vi "Read Image.vi"(8 "error in (no error)":errorcluster, 11 "_Popup in":refnum<class "Popup.lvclass">) -> (0 "error out":errorcluster, 2 "Image":picture, 3 "_Popup out":refnum<class "Popup.lvclass">)   [LabVIEW 2021, in "Pop-Up.lvlib" / "Popup.lvclass"]
doc: "This Data Member Access VI will read the Image from the object.\n\nOutputs: +\n-Image [2D Image] - the image to display on the pop up\n\n<b>Code Developed By:</b> +\nDaniel Coons +\nhttps://github.com/danielcoons/tsc-pop-up"
uses:
  Popup.lvclass
  Popup.lvclass/Popup.ctl
panel:
  # "This VI gets the Image value (PNG graphic) from the Popup Object"
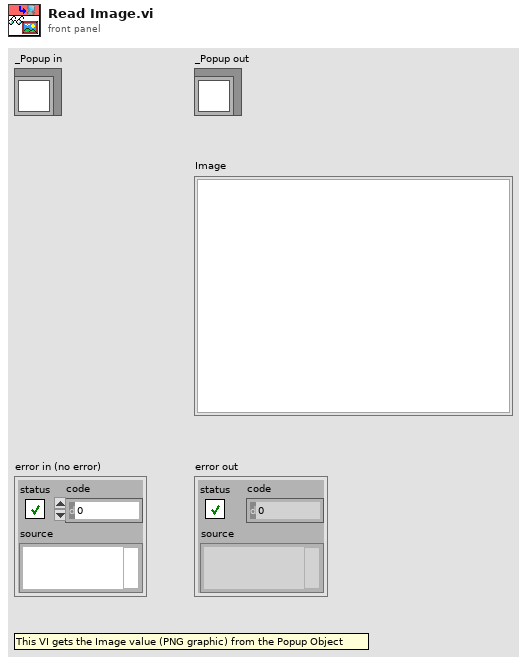
[diagram p1: front panel]
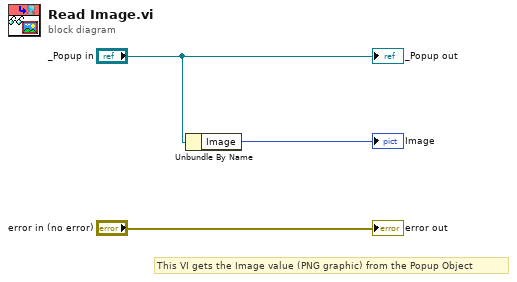
[diagram p0: block diagram]
diagram:
  # "This VI gets the Image value (PNG graphic) from the Popup Object"
  n1 = Unbundle By Name("_Popup in") -> ("Image"=→"Image":picture)
  "error out" <- "error in (no error)"
  "_Popup out" <- "_Popup in"
